vi "Get Data.vi"(8 "error in (no error)":errorcluster, 11 "DataGrid.lvlib:Abstract EVENT.lvclass":refnum<class "Abstract EVENT.lvclass">) -> (0 "error out":errorcluster, 1 "column":i32, 2 "row":i32, 3 "cell value":string)   [LabVIEW 2016, in "DataGrid.lvlib" / "CellValueChanged.lvclass"]
doc: "Converts the class data for cellValue into individual components of the grid"
uses:
  <userlib>/LabVIEWdotNetDataGrid/source/Events/CellValueChanged/CellValueChanged.lvclass
  <userlib>/LabVIEWdotNetDataGrid/source/Events/Abstract EVENT/Abstract EVENT.lvclass
  <userlib>/LabVIEWdotNetDataGrid/source/Events/CellValueChanged/CellValueChanged.lvclass/CellValueChanged.ctl
  <userlib>/LabVIEWdotNetDataGrid/source/Events/CellValueChanged/Read cell value.vi
  <userlib>/LabVIEWdotNetDataGrid/source/Events/CellValueChanged/Read column.vi
  <userlib>/LabVIEWdotNetDataGrid/source/Events/CellValueChanged/Read row.vi
  <vilib>/Utility/error.llb/Error Cluster From Error Code.vi
  <vilib>/ErrorRing/Error Ring.xnode
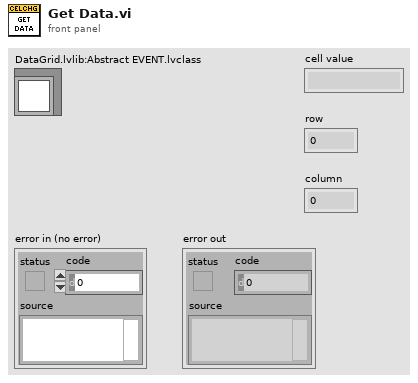
[diagram p1: front panel]
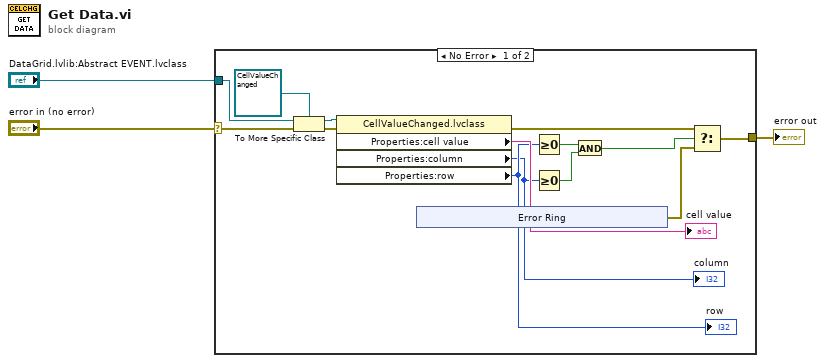
[diagram p0: block diagram]
diagram:
  n1 = case shown="No Error" "error in (no error)" {
    selector: "error in (no error)" -> [w13 w22]
    tunnel: [w5 w22] -> w2
    tunnel: "DataGrid.lvlib:Abstract EVENT.lvclass" -> [w15 _]
    frame No Error {
      n2 = To More Specific Class(target class=refnum<class "CellValueChanged.lvclass"> refnum ("DataGrid.lvlib:CellValueChanged.lvclass"), reference=w15, error in=w13) -> (specific class reference=w14:refnum<class "CellValueChanged.lvclass">, error out=w12:errorcluster)
      n3 = property class="CellValueChanged.lvclass"(reference=w14, error in=w12) -> (error out=w6:errorcluster, "Properties:cell value"=→"cell value":string, "Properties:column"=w10:i32, "Properties:row"=w11:i32)  [unwired: 1 out]
      "column" <- w10
      "row" <- w11
      n4 = xnode "Error Ring"() -> ("error out"=w4:errorcluster)
      n5 = Greater Or Equal To 0?(x=w11) -> (x >= 0?=w9:bool)
      n6 = Greater Or Equal To 0?(x=w10) -> (x >= 0?=w8:bool)
      n7 = And(x=w9, y=w8) -> (x .and. y?=w7:bool)
      n8 = Select(t=w6, s=w7, f=w4) -> (s? t:f=w5:errorcluster)
    }
    frame Error {
    }
  }
  "error out" <- w2
